vi "File.List Subdirs, Sort.vi"(6 "Pattern":string, 8 "error in (no error)":errorcluster, 9 "Order a-z(F), z-a(T)":bool, 10 "Sort Alphabetically":bool, 11 "Dir":path) -> (0 "error out":errorcluster, 1 "Not Empty":bool, 2 "Count":i32, 3 "SubDirs":path[](array[path]))   [LabVIEW 2024]
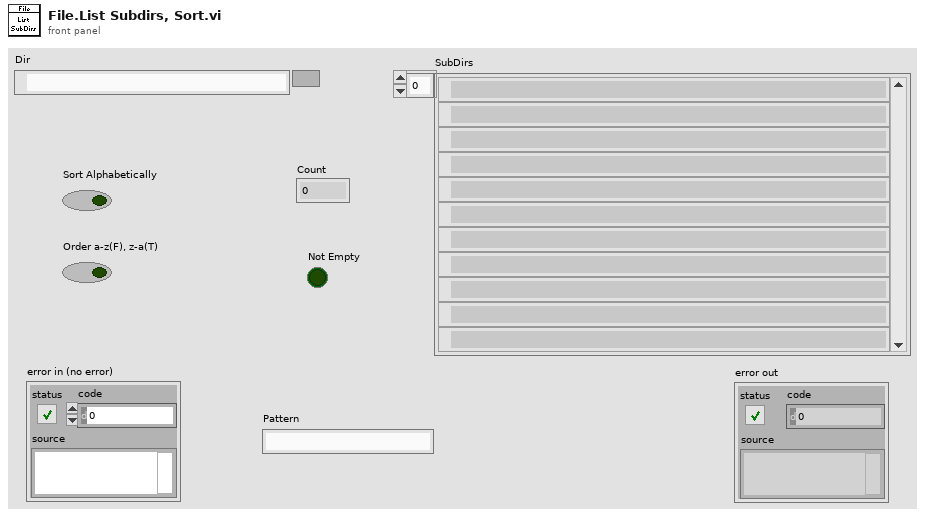
[diagram p1: front panel]
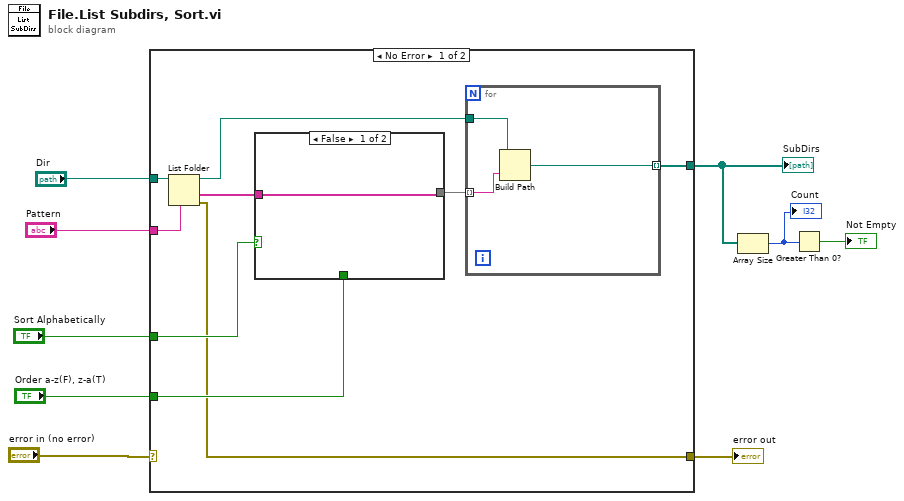
[diagram p0: block diagram]
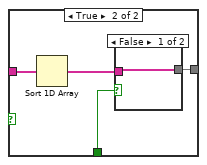
[diagram p2: hidden frame]
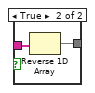
[diagram p3: hidden frame]
diagram:
  n1 = case shown="No Error" "error in (no error)" {
    selector: "error in (no error)" -> [_ w30]
    tunnel: "Dir" -> [w18 _]
    tunnel: [w14 _] -> w3
    tunnel: "Order a-z(F), z-a(T)" -> [w13 _]
    tunnel: "Sort Alphabetically" -> [w12 _]
    tunnel: [w11 w30] -> w5
    tunnel: "Pattern" -> [w10 _]
    frame No Error {
      n2 = List Folder(path=w18, pattern=w10) -> (path out=w15:path, folder names=w17:string[], error out=w11:errorcluster)  [unwired: 2 in, 1 out]
      n3 = case shown="False" w12 {
        tunnel: w17 -> [w19 w23]
        tunnel: [w19 w21] -> w16
        tunnel: w13 -> [_ w20]
        frame False {
        }
        frame True {
          n4 = Sort 1D Array(array=w23) -> (sorted array=w22:string[])
          n5 = case shown="False" w20 {
            tunnel: w22 -> [w24 w26]
            tunnel: [w24 w25] -> w21
            frame False {
            }
            frame True {
              n6 = Reverse 1D Array(array=w26) -> (reversed array=w25:string[])
            }
          }
        }
      }
      n7 = for {
        tunnel: w16 -> [w28] mode=indexing
        tunnel: w15 -> [w29]
        tunnel: [w27] -> w14 mode=indexing
        n8 = Build Path(base path=w29, name or relative path=w28) -> (appended path=w27:path)
      }
    }
    frame Error {
    }
  }
  "SubDirs" <- w3
  "error out" <- w5
  n9 = Array Size(array=w3) -> (size(s)=w1:i32)
  "Count" <- w1
  n10 = Greater Than 0?(x=w1) -> (x > 0?=→"Not Empty":bool)
